vi "Cascaded RC Filter Coefficients.vi"(8 "filter order":i32, 10 "Time Constant":dbl, 11 "Sample rate (Hz)":dbl) -> (1 "Forward Coefficients":dbl[](array[numeric]), 2 "Reverse Coefficients":dbl[](array[numeric]), 3 "IIR Filter Cluster":T1)   [LabVIEW 2019, in "DSP.lvclass"]
uses:
  DSP.lvclass
panel:
  out "concatenated string":string
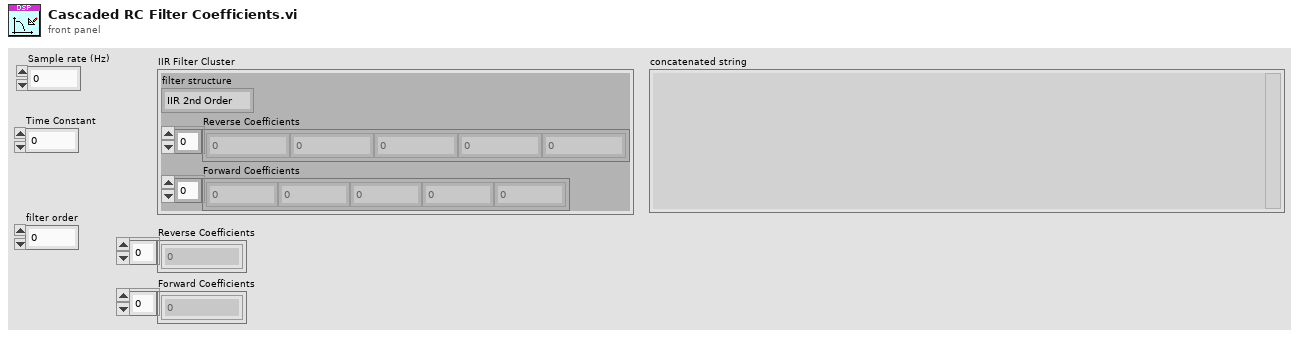
[diagram p1: front panel]
types:
  T1 = cluster{"filter structure":enum32{"IIR 2nd Order", "IIR 4th Order"}, "Reverse Coefficients":dbl[], "Forward Coefficients":dbl[]}
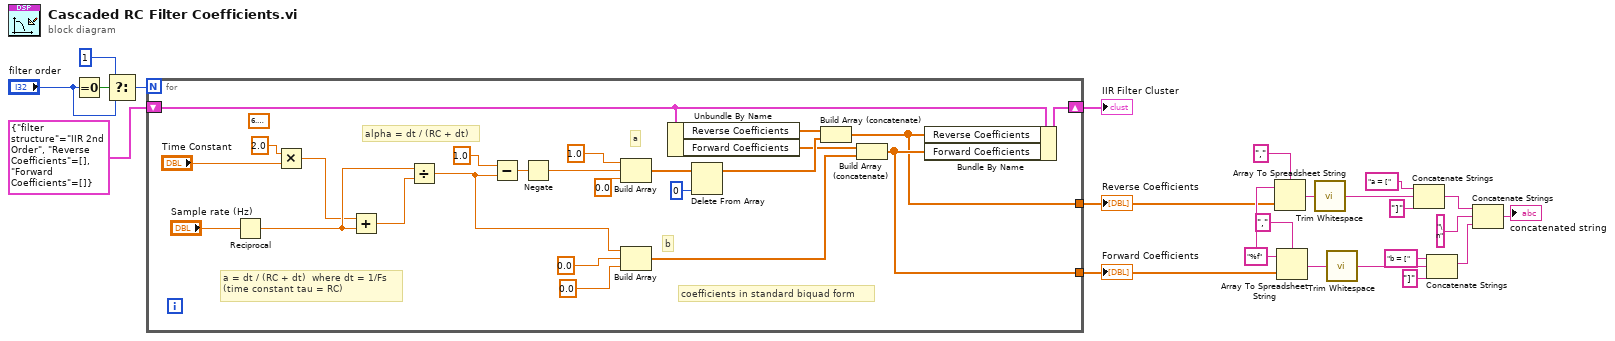
[diagram p0: block diagram]
diagram:
  w9 = "%f" ("format string")
  n1 = Equal To 0?(x="filter order") -> (x = 0?=w23:bool)
  n2 = Select(t=1, s=w23, f="filter order") -> (s? t:f=w21:i32)
  n3 = for {
    N: w21 -> [_]
    shift-right: [w41] -> w18
    shift-left: T1 {"filter structure"=enum."IIR 2nd Order", "Reverse Coefficients"=[], "Forward Coefficients"=[]} ("IIR Filter Cluster") -> [w42]
    tunnel: [w38] -> w2
    tunnel: [w37] -> w3
    (unwired) 6.283185307179586
    # "coefficients in standard biquad form"
    # "alpha = dt / (RC + dt)"
    # "a = dt / (RC + dt)  where dt = 1/Fs\n(time constant tau = RC)"
    # "a"
    # "b"
    n4 = Reciprocal(x="Sample rate (Hz)") -> (1/x=w34:dbl)
    n5 = Multiply(x=2.0 ("y"), y="Time Constant") -> (x*y=w31:dbl)
    n6 = Add(x=w31, y=w34) -> (x+y=w36:dbl)
    n7 = Divide(x=w34, y=w36) -> (x/y=w24:dbl)
    n8 = Subtract(x=1.0 ("y"), y=w24) -> (x-y=w27:dbl)
    n9 = Negate(x=w27) -> (-x=w25:dbl)
    n10 = Build Array(1.0 ("element"), w25, 0.0 ("element")) -> (w46:dbl[])
    n11 = Build Array(w24, 0.0 ("element"), 0.0 ("element")) -> (w39:dbl[])
    n12 = Unbundle By Name(w42) -> ("Reverse Coefficients"=w40:dbl[], "Forward Coefficients"=w43:dbl[])
    n13 = Delete From Array(array=w46, index=0) -> (array with subset deleted=w44:dbl[])  [unwired: 1 in, 1 out]
    n14 = Build Array (concatenate)(w40, w44) -> (w37:dbl[])
    n15 = Build Array (concatenate)(w43, w39) -> (w38:dbl[])
    n16 = Bundle By Name(cluster=w42, "Reverse Coefficients"=w37, "Forward Coefficients"=w38) -> (w41:T1)
  }
  "IIR Filter Cluster" <- w18
  "Reverse Coefficients" <- w3
  "Forward Coefficients" <- w2
  n17 = Array To Spreadsheet String(delimiter (Tab)=",", array=w3, 3:w9) -> (spreadsheet string=w15:string)
  n18 = Array To Spreadsheet String(delimiter (Tab)=",", array=w2, 3:w9) -> (spreadsheet string=w10:string)
  n19 = call <vilib>:"Trim Whitespace.vi"("string"=w15) -> ("trimmed string"=w5:string)  [unwired: 1 in]
  n20 = call <vilib>:"Trim Whitespace.vi"("string"=w10) -> ("trimmed string"=w4:string)  [unwired: 1 in]
  n21 = Concatenate Strings("a = [" ("string"), w5, "]" ("string")) -> (w8:string)
  n22 = Concatenate Strings("b = [" ("string"), w4, "]" ("string")) -> (w7:string)
  n23 = Concatenate Strings(w8, "\n" ("string"), w7) -> (→"concatenated string":string)
